vi "shock_test.vi"() -> ()   [LabVIEW 2024]
uses:
  <vilib>/DAQmx/read.llb/DAQmx Read (Analog 1D Wfm NChan NSamp).vi
  <vilib>/DAQmx/create/channels.llb/DAQmx Create Channel (AI-Voltage-Basic).vi
  <vilib>/DAQmx/create/channels.llb/DAQmx Create Channel (AI-Acceleration-Accelerometer).vi
  <vilib>/DAQmx/configure/timing.llb/DAQmx Timing (Sample Clock).vi
  <vilib>/express/express analysis/Spectral/Block/exnSpectralBlock spectral measurements RMS poly.vi
  <vilib>/express/express analysis/Spectral/Block/exnSpectralBlock spectral measurements RMS WFM.vi
  <vilib>/DAQmx/miscellaneous.llb/DAQmx Fill In Error Info.vi
  <vilib>/express/express analysis/Spectral/Block/exnSpectralBlock spectral measurements RMS DDT.vi
  <vilib>/Utility/file.llb/Write Delimited Spreadsheet (DBL).vi
  <vilib>/express/express analysis/Spectral/XNode/ExpressSpectralMeasurementsBlockNode.xnode
  <resource>/objmgr/daqmx.rc
  <vilib>/measure/NI_MAPro.lvlib
panel:
  out "Array":dbl[](array[numeric])
  in  "Numeric 2":dbl
  in  "Numeric 3":dbl
  out "error out 3":errorcluster
  in  "delimiter (\\t)":string="\t"
  in  "transpose? (no:F)":bool
  in  "error in (no error) 3":errorcluster
  in  "filename 4":path
  out "Filename Out 4":path caption="Filename Out"
  in  "filename 3":path
  out "Filename Out 3":path caption="Filename Out"
  out "AO_output_acc":waveform(dbl)(graph)
  out "AO_input_acc":waveform(dbl)(graph)
  out "AO_Voltage":waveform(dbl)(graph)
  out "FFT magnitude 3":dynamicdata(graph)
  out "ACC Time domain 3":dynamicdata(graph)
  out "VOLT Time domain 2":dynamicdata(graph)
  out "FFT magnitude 2":dynamicdata(graph)
  out "error out 2":errorcluster
  in  "error in (no error) 2":errorcluster
  in  "sampling info 2":cluster{"Fs":dbl, "#s":dbl}={"Fs"=1000.0, "#s"=1000.0} {"Fs" format="%.2p"}
  in  "frequency 2":dbl=10.0 format="%0.2p"
  in  "amplitude 2":dbl=1.0 format="%0.2p"
  in  "formula 2":string="sin(w*t)*sin(2*pi(1)*t)"
  out "Waveform Graph 4":waveform(dbl)(graph)
  out "error out":errorcluster
  in  "error in (no error)":errorcluster
  in  "sampling info":cluster{"Fs":dbl, "#s":dbl}={"Fs"=1000.0, "#s"=1000.0} {"Fs" format="%.2p"}
  in  "frequency":dbl=10.0 format="%0.2p"
  in  "amplitude":dbl=1.0 format="%0.2p"
  in  "formula":string="sin(w*t)*sin(2*pi(1)*t)"
  out "Waveform Graph 3":waveform(dbl)(graph)
  out "end index":i32
  out "start index":i32
  in  "end time":dbl
  in  "start time":dbl
  out "FFT excitation":cluster{"f0":dbl, "df":dbl, "magnitude":dbl[]}(graph)
  in  "voltage scale":dbl
  in  "output frequency":dbl
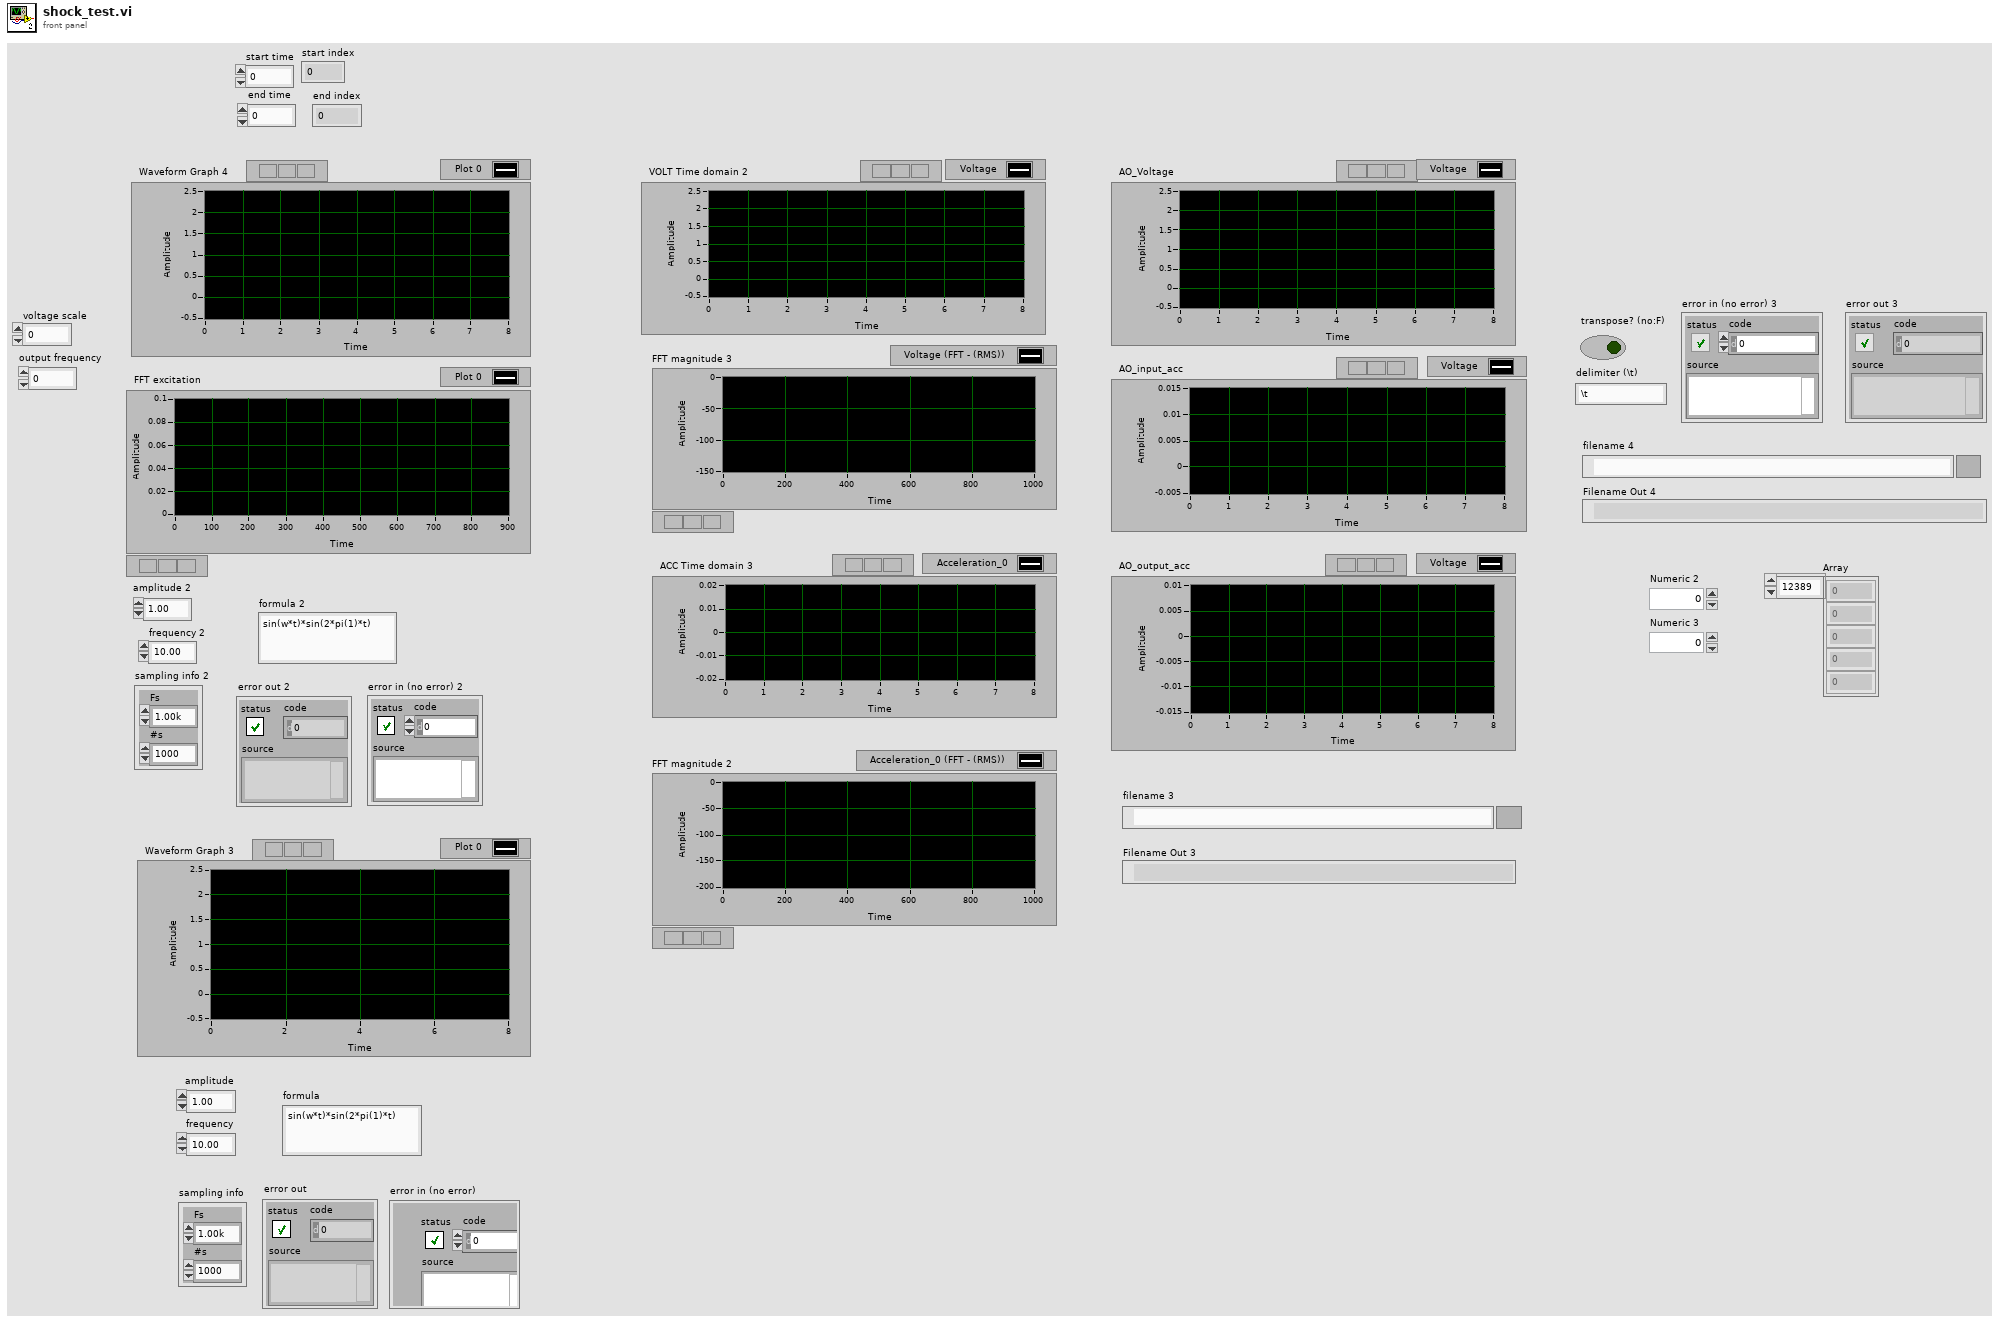
[diagram p1: front panel]
types:
  T1 = cluster{"averaging mode":u16, "weighting mode":u16, "number of averages":u32}
  T2 = cluster{"dB On (F)":bool, "unwrap phase (F)":bool, "convert to degree (F)":bool}
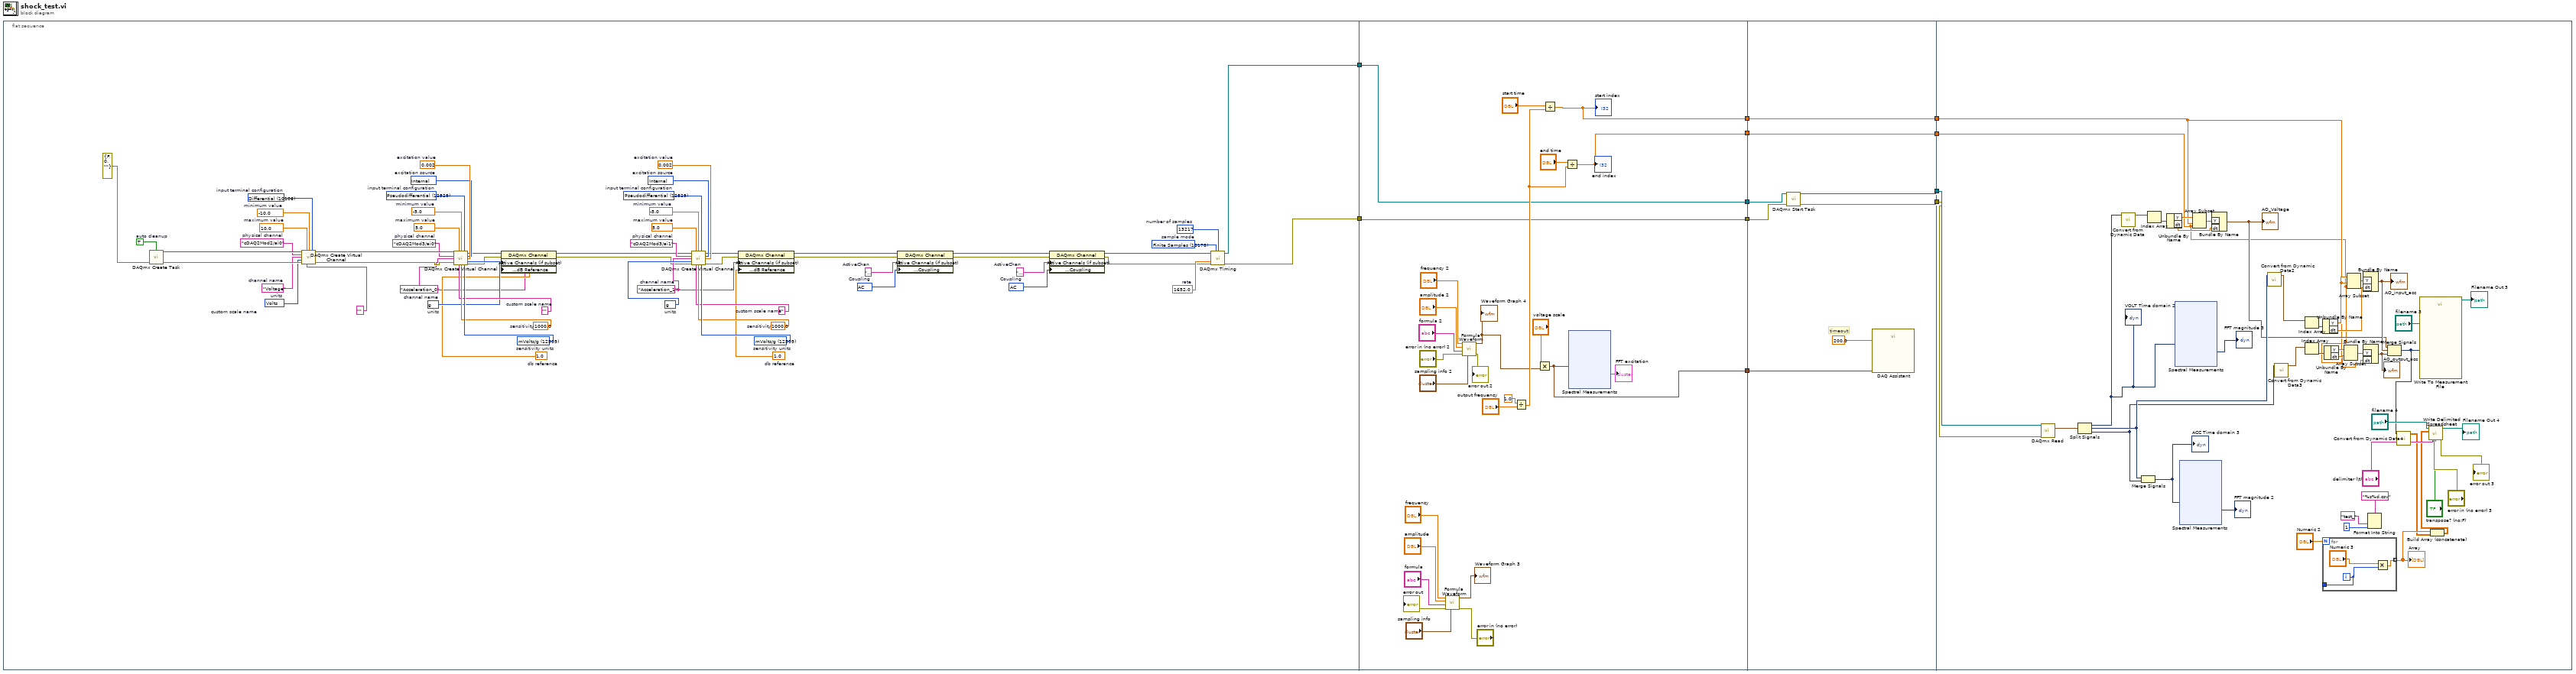
[diagram p0: block diagram]
diagram:
  n1 = flat-sequence {
    tunnel: [w13] -> w11
    tunnel: [w12] -> w7
    tunnel: w11 -> [w73]
    tunnel: [w74] -> w10
    tunnel: [w73] -> w9
    tunnel: [w72] -> w8
    tunnel: w7 -> [w72]
    tunnel: [w71] -> w3
    tunnel: [w70] -> w1
    tunnel: w10 -> [w112]
    tunnel: w9 -> [w111]
    tunnel: w8 -> [w110]
    tunnel: [w109] -> w6
    tunnel: [w108] -> w5
    tunnel: [w107] -> w4
    tunnel: w3 -> [w107]
    tunnel: [w106] -> w2
    tunnel: w1 -> [w106]
    tunnel: w6 -> [w115]
    tunnel: w5 -> [w114]
    tunnel: w4 -> [w117]
    tunnel: w2 -> [w116]
    frame #0 {
      w59 = 10106 items=["default"=-1, "RSE"=10083, "NRSE"=10078, "Differential"=10106, "Pseudodifferential"=12529]  # input terminal configuration
      w60 = 10348 items=["Volts"=10348, "From Custom Scale"=10065]  # units
      w61 = "Voltage"  # channel name
      w62 = ""  # custom scale name
      w63 = -10.0  # minimum value
      w64 = 10.0  # maximum value
      w65 = "cDAQ2Mod2/ai0"  # physical channel
      w26 = 10178 items=["Finite Samples"=10178, "Continuous Samples"=10123, "Hardware Timed Single Point"=12522]  # sample mode
      w27 = 13217  # number of samples
      w28 = 1652.0  # rate
      w30 = 10045 items=["AC"=10045, "DC"=10050, "GND"=10066]  # Coupling
      w29 = "Acceleration_1"  # ActiveChan
      w32 = 10045 items=["AC"=10045, "DC"=10050, "GND"=10066]  # Coupling
      w31 = "Acceleration_0"  # ActiveChan
      w34 = 1.0  # db reference
      w41 = 10186 items=["g"=10186, "m/s^2"=12470, "From Custom Scale"=10065]  # units
      w37 = 12529 items=["default"=-1, "RSE"=10083, "NRSE"=10078, "Differential"=10106, "Pseudodifferential"=12529]  # input terminal configuration
      w39 = 10200 items=["Internal"=10200, "External"=10167, "None"=10230]  # excitation source
      w40 = 0.002  # excitation value
      w44 = 12509 items=["mVolts/g"=12509, "Volts/g"=12510]  # sensitivity units
      w43 = 1000.0  # sensitivity
      w33 = "Acceleration_1"  # channel name
      w42 = ""  # custom scale name
      w36 = -5.0  # minimum value
      w35 = 5.0  # maximum value
      w38 = "cDAQ2Mod3/ai1"  # physical channel
      w46 = 1.0  # db reference
      w53 = 10186 items=["g"=10186, "m/s^2"=12470, "From Custom Scale"=10065]  # units
      w49 = 12529 items=["default"=-1, "RSE"=10083, "NRSE"=10078, "Differential"=10106, "Pseudodifferential"=12529]  # input terminal configuration
      w51 = 10200 items=["Internal"=10200, "External"=10167, "None"=10230]  # excitation source
      w52 = 0.002  # excitation value
      w56 = 12509 items=["mVolts/g"=12509, "Volts/g"=12510]  # sensitivity units
      w55 = 1000.0  # sensitivity
      w45 = "Acceleration_0"  # channel name
      w54 = ""  # custom scale name
      w48 = -5.0  # minimum value
      w47 = 5.0  # maximum value
      w50 = "cDAQ2Mod3/ai0"  # physical channel
      w57 = TRUE  # auto cleanup
      n2 = call <vilib>:"DAQmx Create Task.vi"("auto cleanup"=w57, "error in"=errorcluster {"status"=FALSE, "code"=0, "source"=""}) -> ("task out"=w66:refnum<k21>, "error out"=w67:errorcluster)  [unwired: 12 in]
      n3 = call-poly <vilib>:"DAQmx Create Virtual Channel.vi"("task in"=w66, "maximum value"=w64, "minimum value"=w63, "input terminal configuration"=w59, "physical channels"=w65, "name to assign"=w61, "units"=w60, "error in"=w67, "custom scale name"=w62) -> ("task out"=w68:refnum<k21>, "error out"=w69:errorcluster)  [unwired: 5 in]
      n4 = call-poly <vilib>:"DAQmx Create Virtual Channel.vi"("task in"=w68, "maximum value"=w47, "minimum value"=w48, "input terminal configuration"=w49, "physical channels"=w50, "current excitation source"=w51, "name to assign"=w45, "current excitation value"=w52, "units"=w53, "error in"=w69, "custom scale name"=w54, "sensitivity"=w55, "sensitivity units"=w56) -> ("task out"=w14:refnum<k21>, "error out"=w15:errorcluster)  [unwired: 1 in]
      n5 = property class="DAQmx Channel"(reference=w14, error in=w15, "Active Channels (if subset)"=w45, "Analog Input:Acceleration:dB Reference"=w46) -> (reference out=w17:refnum<k21>, error out=w16:errorcluster)
      n6 = call-poly <vilib>:"DAQmx Create Virtual Channel.vi"("task in"=w17, "maximum value"=w35, "minimum value"=w36, "input terminal configuration"=w37, "physical channels"=w38, "current excitation source"=w39, "name to assign"=w33, "current excitation value"=w40, "units"=w41, "error in"=w16, "custom scale name"=w42, "sensitivity"=w43, "sensitivity units"=w44) -> ("task out"=w18:refnum<k21>, "error out"=w19:errorcluster)  [unwired: 1 in]
      n7 = property class="DAQmx Channel"(reference=w18, error in=w19, "Active Channels (if subset)"=w33, "Analog Input:Acceleration:dB Reference"=w34) -> (reference out=w22:refnum<k21>, error out=w20:errorcluster)
      n8 = property class="DAQmx Channel"(reference=w22, error in=w20, "Active Channels (if subset)"=w31, "Analog Input:General Properties:Input Configuration:Coupling"=w32) -> (reference out=w24:refnum<k21>, error out=w21:errorcluster)
      n9 = property class="DAQmx Channel"(reference=w24, error in=w21, "Active Channels (if subset)"=w29, "Analog Input:General Properties:Input Configuration:Coupling"=w30) -> (reference out=w25:refnum<k21>, error out=w23:errorcluster)
      n10 = call-poly <vilib>:"DAQmx Timing.vi"("task/channels in"=w25, "sample mode"=w26, "samples per channel"=w27, "rate"=w28, "error in"=w23) -> ("task out"=w13:refnum<k21>, "error out"=w12:errorcluster)  [unwired: 9 in]
    }
    frame #1 {
      n11 = call <vilib>:"Formula Waveform.vi"("sampling info"="sampling info", "error in (no error)"="error in (no error)", "formula"="formula", "amplitude"="amplitude", "frequency"="frequency") -> ("error out"=→"error out":errorcluster, "signal out"=→"Waveform Graph 3":waveform(dbl))  [unwired: 5 in]
      n12 = call <vilib>:"Formula Waveform.vi"("sampling info"="sampling info 2", "error in (no error)"="error in (no error) 2", "formula"="formula 2", "amplitude"="amplitude 2", "frequency"="frequency 2") -> ("error out"=→"error out 2":errorcluster, "signal out"=w76:waveform(dbl))  [unwired: 5 in]
      "Waveform Graph 4" <- w76
      n13 = Divide(x=1.0, y="output frequency") -> (x/y=w90:dbl)
      n14 = Multiply(x="voltage scale", y=w76) -> (x*y=w74:waveform(dbl))
      n15 = Divide(x="start time", y=w90) -> (x/y=w71:dbl)
      "start index" <- w71
      n16 = Divide(x="end time", y=w90) -> (x/y=w70:dbl)
      "end index" <- w70
      n17 = xnode "Spectral Measurements"("Signals"=w74) -> ("FFT - (RMS)"=→"FFT excitation":cluster{"f0":dbl, "df":dbl, "magnitude":dbl[]})  [unwired: 1 in, 2 out]
    }
    frame #2 {
      # "timeout"
      n18 = call <vilib>:"DAQmx Start Task.vi"("task/channels in"=w111, "error in"=w110) -> ("task out"=w109:refnum<k21>, "error out"=w108:errorcluster)  [unwired: 12 in]
      n19 = call "DAQ Assistant"("data"=w112, "timeout (s)"=200.0) -> ()  [unwired: 16 in, 2 out]
    }
    frame #3 {
      n20 = call-poly <vilib>:"DAQmx Read.vi"("task/channels in"=w115, "error in"=w114) -> ("data"=w156:waveform(dbl)[])  [unwired: 11 in, 2 out]
      n21 = Split Signals(w156) -> (w155:dynamicdata, w137:dynamicdata, w136:dynamicdata)  [unwired: 3 in]
      "VOLT Time domain 2" <- w155
      n22 = call "Convert from Dynamic Data"("Dynamic Data Type"=w155) -> ("Array of Waveform"=w154:waveform(dbl)[])  [unwired: 3 in]
      n23 = Merge Signals(w137, w136) -> (w133:dynamicdata)
      "ACC Time domain 3" <- w133
      n24 = Index Array(array=w154) -> (element=w153:waveform(dbl))  [unwired: 1 in]
      n25 = Unbundle By Name(w153) -> ("Y"=w152:dbl[], "dt"=w151:dbl)
      n26 = xnode "Spectral Measurements"("Signals"=w155) -> ("FFT - (RMS)"=→"FFT magnitude 3":dynamicdata)  [unwired: 1 in, 2 out]
      n27 = xnode "Spectral Measurements"("Signals"=w133) -> ("FFT - (RMS)"=→"FFT magnitude 2":dynamicdata)  [unwired: 1 in, 2 out]
      n28 = Array Subset(array=w152, index=w117, length=w116) -> (w150:dbl[])
      n29 = Bundle By Name("Y"=w150, "dt"=w151) -> (w134:waveform(dbl))  [unwired: 1 in]
      "AO_Voltage" <- w134
      n30 = call "Convert from Dynamic Data2"("Dynamic Data Type"=w137) -> ("Array of Waveform"=w149:waveform(dbl)[])  [unwired: 3 in]
      n31 = call "Convert from Dynamic Data3"("Dynamic Data Type"=w136) -> ("Array of Waveform"=w144:waveform(dbl)[])  [unwired: 3 in]
      n32 = Index Array(array=w149) -> (element=w148:waveform(dbl))  [unwired: 1 in]
      n33 = Index Array(array=w144) -> (element=w143:waveform(dbl))  [unwired: 1 in]
      n34 = Unbundle By Name(w148) -> ("Y"=w147:dbl[], "dt"=w146:dbl)
      n35 = for {
        N: "Numeric 2" -> [_]
        tunnel: [w161] -> _
        tunnel: [w159] -> w125 mode=indexing
        i -> [w161]
        n36 = Multiply(x="Numeric 3", y=w161) -> (x*y=w159:dbl)
      }
      "Array" <- w125
      n37 = Unbundle By Name(w143) -> ("Y"=w142:dbl[], "dt"=w127:dbl)
      n38 = Array Subset(array=w142, index=w117, length=w116) -> (w141:dbl[])
      n39 = Array Subset(array=w147, index=w117, length=w116) -> (w145:dbl[])
      n40 = Bundle By Name("Y"=w145, "dt"=w146) -> (w135:waveform(dbl))  [unwired: 1 in]
      "AO_input_acc" <- w135
      n41 = Bundle By Name("Y"=w141, "dt"=w127) -> (w140:waveform(dbl))  [unwired: 1 in]
      "AO_output_acc" <- w140
      n42 = Format Into String(format string="%s%d.csv", "test_", 1) -> ()  [unwired: 2 in, 2 out]
      n43 = Merge Signals(w134, w135, w140) -> (w119:dynamicdata)
      n44 = call "Convert from Dynamic Data4"("Dynamic Data Type"=w119) -> ("Array"=w118:dbl[][])  [unwired: 3 in]
      n45 = call "Write To Measurement File"("Signals"=w119, "Filename"="filename 3") -> ("Filename Out"=→"Filename Out 3":path)  [unwired: 15 in, 2 out]
      n46 = Build Array (concatenate)(w125, w118) -> (w124:dbl[][])
      n47 = call-poly <vilib>:"Write Delimited Spreadsheet.vi"("file path (dialog if empty)"="filename 4", "2D data"=w124, "error in (no error)"="error in (no error) 3", "transpose? (no:F)"="transpose? (no:F)", "delimiter (\\t)"="delimiter (\\t)") -> ("new file path (Not A Path if cancelled)"=→"Filename Out 4":path, "error out"=→"error out 3":errorcluster)  [unwired: 9 in]
    }
  }
